vi "SaveRunData(SubVI).vi"(0 "Data cluster":T1, 11 "error in (no error)":errorcluster) -> (15 "error out":errorcluster)   [LabVIEW 2020]
doc: "[Covers: REQ1]\n[Covers: REQ3]\nSave data file as tdms"
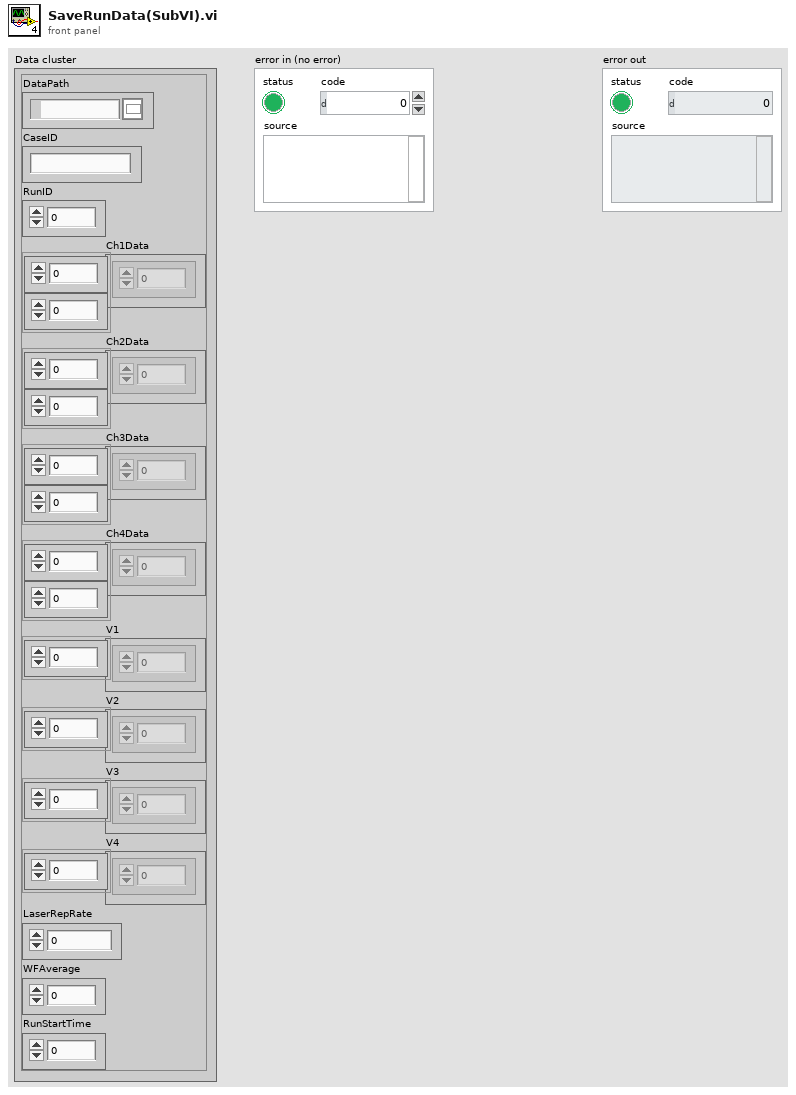
[diagram p1: front panel]
types:
  T1 = cluster{"DataPath":path, "CaseID":string, "RunID":i16, "Ch1Data":dbl[][], "Ch2Data":dbl[][], "Ch3Data":dbl[][], "Ch4Data":dbl[][], "V1":dbl[], "V2":dbl[], "V3":dbl[], "V4":dbl[], "LaserRepRate":u16, "WFAverage":i16, "RunStartTime":u64}
  T2 = enum16{"open", "open or create", "create or replace", "create", "open (read-only)"}
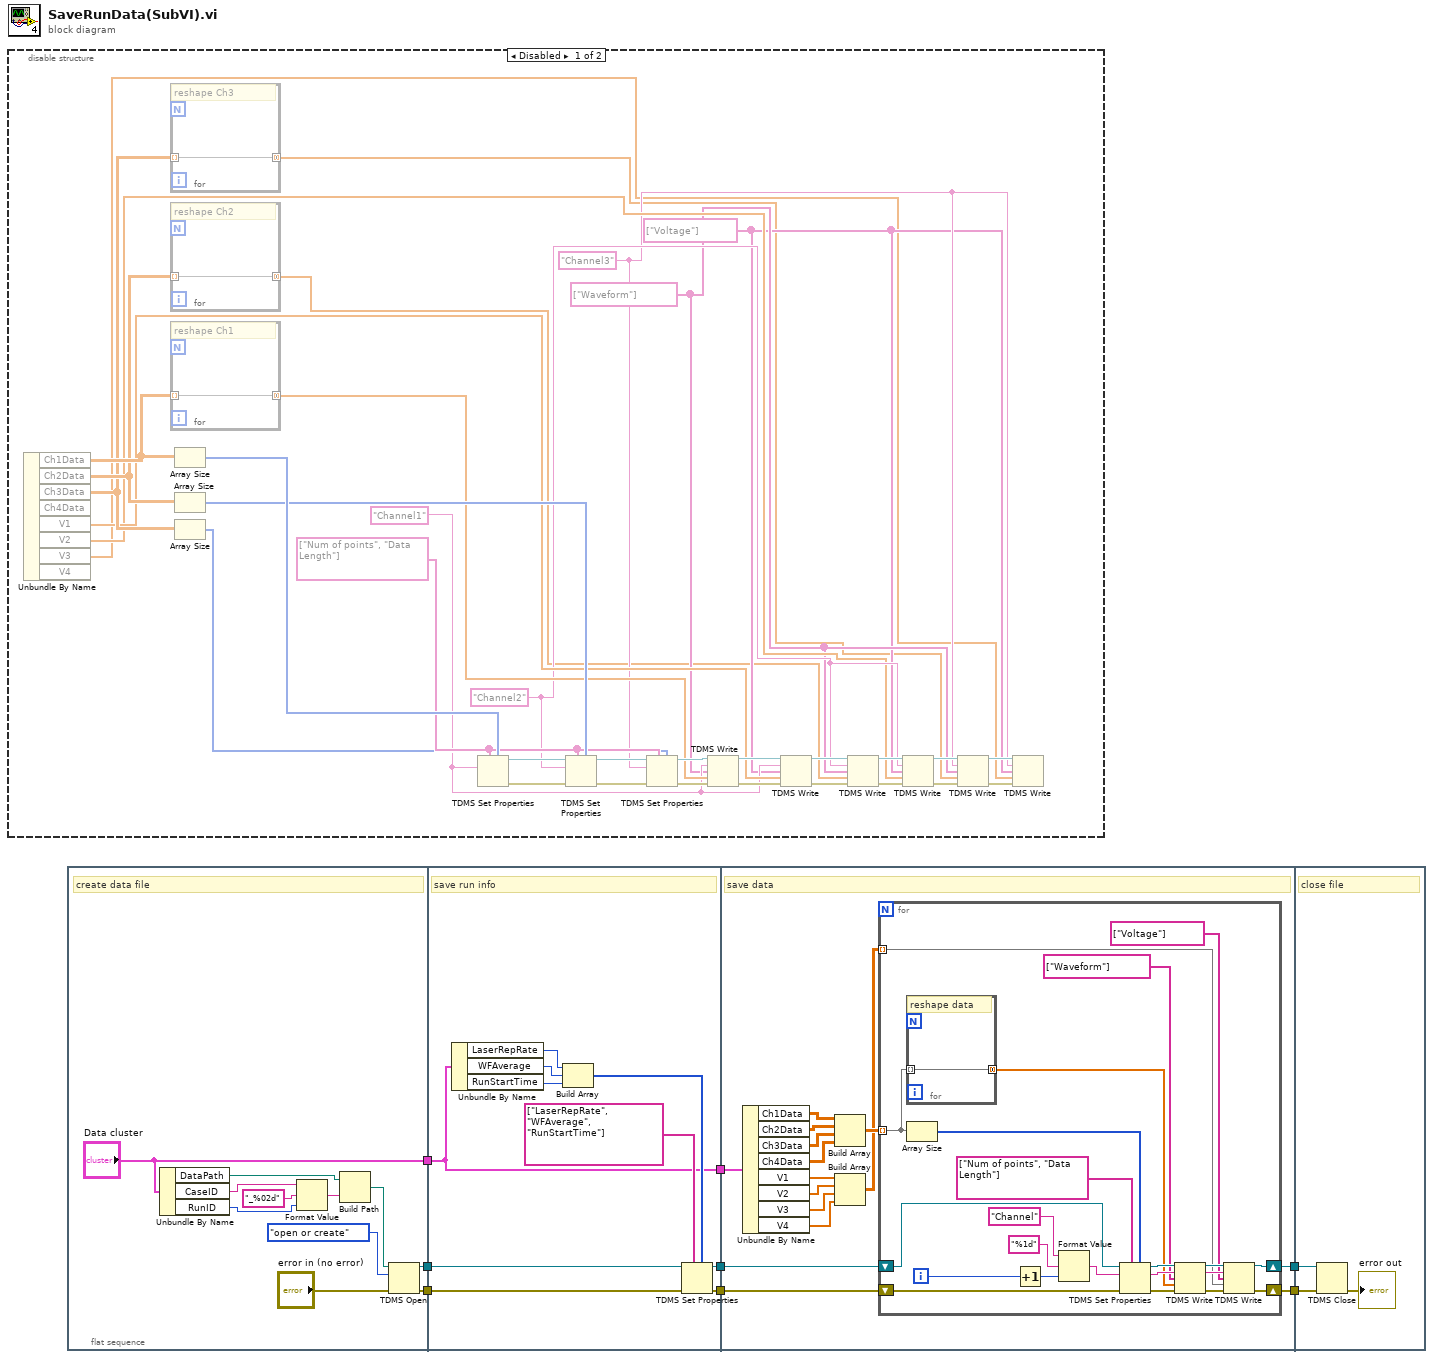
[diagram p0: block diagram]
diagram:
  n1 = disable-structure shown="Disabled" {
    frame Disabled {
      w12 = string[] ["Voltage"] ("channel name(s) in (Untitled)")
      w13 = string[] ["Waveform"] ("channel name(s) in (Untitled)")
      w14 = "Channel3" ("group name")
      w16 = "Channel2" ("group name")
      w25 = string[] ["Num of points", "Data Length"] ("property names")
      w17 = "Channel1" ("group name")
      n2 = Unbundle By Name() -> ("Ch1Data"=w33:dbl[][], "Ch2Data"=w29:dbl[][], "Ch3Data"=w24:dbl[][], "V1"=w18:dbl[], "V2"=w15:dbl[], "V3"=w9:dbl[])  [unwired: 1 in, 2 out]
      n3 = for {
        tunnel: w24 -> [w43] mode=indexing
        tunnel: [w43] -> w10 mode=concatenating
        # "reshape Ch3"
      }
      n4 = for {
        tunnel: w29 -> [w44] mode=indexing
        tunnel: [w44] -> w11 mode=concatenating
        # "reshape Ch2"
      }
      n5 = for {
        tunnel: w33 -> [w45] mode=indexing
        tunnel: [w45] -> w20 mode=concatenating
        # "reshape Ch1"
      }
      n6 = Array Size(array=w33) -> (size(s)=w32:i32[])
      n7 = Array Size(array=w29) -> (size(s)=w28:i32[])
      n8 = Array Size(array=w24) -> (size(s)=w23:i32[])
      n9 = TDMS Set Properties(5:w32, 7:w25, 10:w17) -> (0:w30:errorcluster, 3:w31:refnum<k34>)  [unwired: 3 in, 2 out]
      n10 = TDMS Set Properties(5:w28, 7:w25, 8:w30, 10:w16, 11:w31) -> (0:w26:errorcluster, 3:w27:refnum<k34>)  [unwired: 1 in, 2 out]
      n11 = TDMS Set Properties(5:w23, 7:w25, 8:w26, 10:w14, 11:w27) -> (0:w21:errorcluster, 3:w22:refnum<k34>)  [unwired: 1 in, 2 out]
      n12 = TDMS Write(0:w22, 5:w17, 7:w13, 9:w20, 11:w21) -> (4:w34:refnum<k34>, 15:w19:errorcluster)  [unwired: 1 in, 2 out]
      n13 = TDMS Write(0:w34, 5:w17, 7:w12, 9:w18, 11:w19) -> (4:w35:refnum<k34>, 15:w36:errorcluster)  [unwired: 1 in, 2 out]
      n14 = TDMS Write(0:w35, 5:w16, 7:w13, 9:w11, 11:w36) -> (4:w37:refnum<k34>, 15:w38:errorcluster)  [unwired: 1 in, 2 out]
      n15 = TDMS Write(0:w37, 5:w16, 7:w12, 9:w15, 11:w38) -> (4:w42:refnum<k34>, 15:w39:errorcluster)  [unwired: 1 in, 2 out]
      n16 = TDMS Write(0:w42, 5:w14, 7:w13, 9:w10, 11:w39) -> (4:w40:refnum<k34>, 15:w41:errorcluster)  [unwired: 1 in, 2 out]
      n17 = TDMS Write(0:w40, 5:w14, 7:w12, 9:w9, 11:w41) -> ()  [unwired: 1 in, 4 out]
    }
    frame Enabled {
    }
  }
  n18 = flat-sequence {
    tunnel: ["Data cluster"] -> w8
    tunnel: [w48] -> w5
    tunnel: [w47] -> w4
    tunnel: w8 -> [w57]
    tunnel: [w65] -> w7
    tunnel: [w64] -> w6
    tunnel: w5 -> [w59]
    tunnel: w4 -> [w58]
    tunnel: [w57] -> w3
    tunnel: w7 -> [w70]
    tunnel: w6 -> [w71]
    tunnel: w3 -> [w81]
    tunnel: [w68] -> w2
    tunnel: [w67] -> w1
    tunnel: w2 -> [w106]
    tunnel: w1 -> [w105]
    frame #0 {
      # "create data file"
      n19 = Unbundle By Name("Data cluster") -> ("DataPath"=w51:path, "CaseID"=w50:string, "RunID"=w49:i16)
      n20 = Format Value(string ("")=w50, format string="_%02d", value (0)=w49) -> (output string=w54:string)
      n21 = Build Path(base path=w51, name or relative path=w54) -> (appended path=w56:path)
      n22 = TDMS Open(8:"error in (no error)", 10:T2."open or create" ("operation (0:open)"), 11:w56) -> (0:w47:errorcluster, 3:w48:refnum<k34>)  [unwired: 4 in]
    }
    frame #1 {
      # "save run info"
      n23 = Unbundle By Name(w57) -> ("LaserRepRate"=w63:u16, "WFAverage"=w62:i16, "RunStartTime"=w61:u64)
      n24 = Build Array(w63, w62, w61) -> (w66:u64[])
      n25 = TDMS Set Properties(5:w66, 7:string[] ["LaserRepRate", "WFAverage", "RunStartTime"] ("property names"), 8:w58, 11:w59) -> (0:w65:errorcluster, 3:w64:refnum<k34>)  [unwired: 2 in, 2 out]
    }
    frame #2 {
      # "save data"
      n26 = Unbundle By Name(w81) -> ("Ch1Data"=w80:dbl[][], "Ch2Data"=w79:dbl[][], "Ch3Data"=w78:dbl[][], "Ch4Data"=w77:dbl[][], "V1"=w75:dbl[], "V2"=w74:dbl[], "V3"=w73:dbl[], "V4"=w72:dbl[])
      n27 = Build Array(w80, w79, w78, w77) -> (w76:dbl[][][])
      n28 = Build Array(w75, w74, w73, w72) -> (w69:dbl[][])
      n29 = for {
        tunnel: w76 -> [w90] mode=indexing
        shift-right: [w83] -> w68
        shift-left: w71 -> [w99]
        shift-right: [w82] -> w67
        shift-left: w70 -> [w98]
        tunnel: w69 -> [w84] mode=indexing
        i -> [w101]
        n30 = for {
          tunnel: w90 -> [w104] mode=indexing
          tunnel: [w104] -> w89 mode=concatenating
          # "reshape data"
        }
        n31 = Array Size(array=w90) -> (size(s)=w95:i32[])
        n32 = Increment(x=w101) -> (x+1=w100:i32)
        n33 = Format Value(string ("")="Channel", format string="%1d", value (0)=w100) -> (output string=w97:string)
        n34 = TDMS Set Properties(5:w95, 7:string[] ["Num of points", "Data Length"] ("property names"), 8:w98, 10:w97, 11:w99) -> (0:w93:errorcluster, 2:w92:string, 3:w94:refnum<k34>)  [unwired: 1 in, 1 out]
        n35 = TDMS Write(0:w94, 5:w92, 7:string[] ["Waveform"] ("channel name(s) in (Untitled)"), 9:w89, 11:w93) -> (4:w88:refnum<k34>, 6:w87:string, 15:w86:errorcluster)  [unwired: 1 in, 1 out]
        n36 = TDMS Write(0:w88, 5:w87, 7:string[] ["Voltage"] ("channel name(s) in (Untitled)"), 9:w84, 11:w86) -> (4:w83:refnum<k34>, 15:w82:errorcluster)  [unwired: 1 in, 2 out]
      }
    }
    frame #3 {
      # "close file"
      n37 = TDMS Close(8:w105, 11:w106) -> (0:→"error out":errorcluster)  [unwired: 1 out]
    }
  }
